vi "ReadChangedFileLogPaths.vi"(8 "error in (no error)":errorcluster, 10 "Workspace Path":path, 11 "Refnum in":T1) -> (0 "error out":errorcluster, 2 "ChangedFilesLogpaths":map{string, path}(c390), 3 "refnum out":T1)   [LabVIEW 2023, in "DepsWatch.lvlib"]
uses:
  DepsWatch.lvlib
  <vilib>/Utility/config.llb/Config Data RefNum.ctl
  <vilib>/Utility/config.llb/Read Key (String).vi
  <vilib>/Utility/config.llb/NI_LVConfig.lvlib
  <userlib>/_OpenG.lib/file/file.llb/openg_file.lvlib
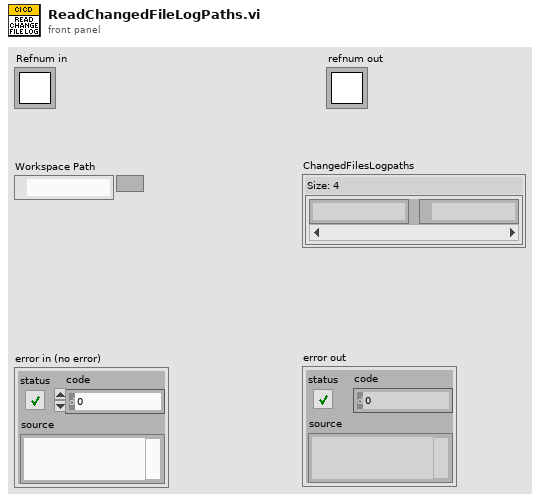
[diagram p1: front panel]
types:
  T1 = typedef "NI_LVConfig.lvlib/Config Data RefNum.ctl" = refnum<k1>
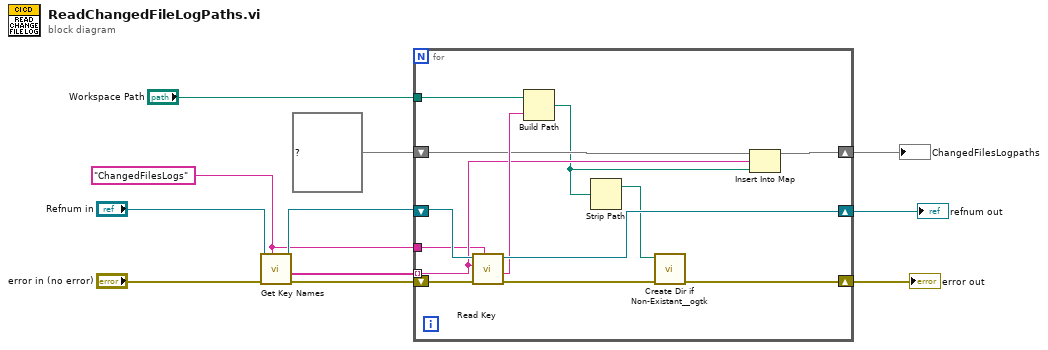
[diagram p0: block diagram]
diagram:
  w1 = "ChangedFilesLogs" ("section")
  n1 = call <vilib>:"Get Key Names.vi"("section"=w1, "error in (no error)"="error in (no error)", "refnum"="Refnum in") -> ("error out"=w9:errorcluster, "key names"=w10:string[], "refnum out"=w8:T1)  [unwired: 5 in, 1 out]
  n2 = for {
    shift-right: [w14] -> w4
    shift-left: w9 -> [w15]
    tunnel: w10 -> [w18] mode=indexing
    tunnel: "Workspace Path" -> [w23]
    shift-right: [w21] -> w5
    shift-left: w8 -> [w22]
    shift-right: [w17] -> w2
    shift-left: map{string, path} {} ("map") -> [w19]
    tunnel: w1 -> [w16]
    n3 = call-poly <vilib>:"Read Key.vi"("section"=w16, "error in (no error)"=w15, "key"=w18, "refnum"=w22) -> ("value"=w20:string, "refnum out"=w21:T1)  [unwired: 4 in, 2 out]
    n4 = Build Path(base path=w23, name or relative path=w20) -> (appended path=w13:path)
    n5 = Strip Path(path=w13) -> (stripped path=w12:path)  [unwired: 1 out]
    n6 = call <userlib>:"Create Dir if Non-Existant__ogtk.vi"("error in (no error)"=w15, "Directory Path"=w12) -> ("error out"=w14:errorcluster)  [unwired: 7 in, 2 out]
    n7 = Insert Into Map(map in=w19, key=w18, value=w13) -> (map out=w17:map{string, path})  [unwired: 2 out]
  }
  "refnum out" <- w5
  "error out" <- w4
  "ChangedFilesLogpaths" <- w2
